vi "LWXPS_GroupReferencingActionExecute.vi"(5 "LabVIEW error IN":errorcluster, 6 "XPS Reference IN":refnum<k24>, 7 "Referencing Parameter":dbl, 8 "Referencing Sensor":string, 9 "Referencing Action":string, 10 "Positioner Name":string) -> (0 "LabVIEW error OUT":errorcluster, 1 "XPS Error String":string, 2 "Returned error code":i32, 3 "XPS Reference OUT":refnum<k24>)   [LabVIEW 2014]
uses:
  D:/XPSQ8_LabView_Library/Development/Source/Dll/Newport.XPS.CommandInterface.dll
  Dll/Newport.XPS.CommandInterface.dll
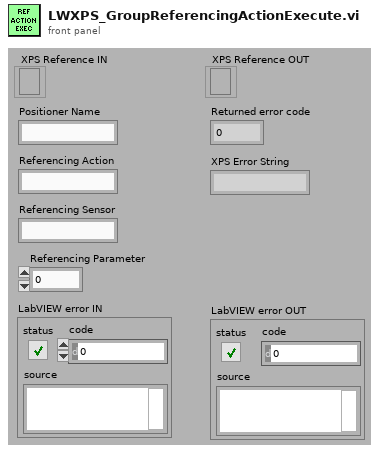
[diagram p1: front panel]
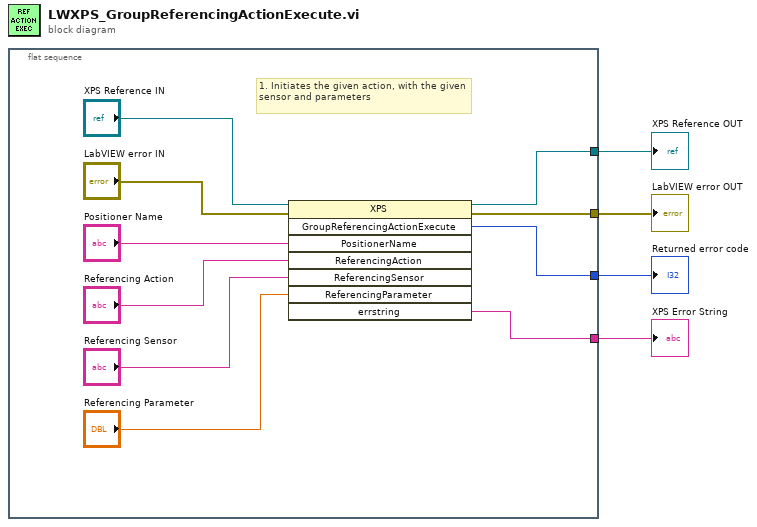
[diagram p0: block diagram]
diagram:
  n1 = flat-sequence {
    tunnel: [w10] -> w4
    tunnel: [w12] -> w3
    tunnel: [w13] -> w2
    tunnel: [w9] -> w1
    frame #0 {
      # "1. Initiates the given action, with the given sensor and parameters"
      n2 = invoke class="XPS" method="GroupReferencingActionExecute"(reference="XPS Reference IN", error in="LabVIEW error IN", "PositionerName"="Positioner Name", "ReferencingAction"="Referencing Action", "ReferencingSensor"="Referencing Sensor", "ReferencingParameter"="Referencing Parameter") -> (reference out=w10:refnum<k24>, error out=w12:errorcluster, "GroupReferencingActionExecute"=w13:i32, "errstring"=w9:string)  [unwired: 2 in, 4 out]
    }
  }
  "XPS Reference OUT" <- w4
  "LabVIEW error OUT" <- w3
  "Returned error code" <- w2
  "XPS Error String" <- w1
